vi "Subpanel PoC.vi"() -> ()   [LabVIEW 2021]
uses:
  <vilib>/Utility/LVLibp/NI_PackedLibraryUtility.lvlib
panel:
  in  "stop":bool
  out "qualified names":string[](array[string])
  out "error out":errorcluster
  in  "vi path":path=path "D:/dev/builds/TemplatePlugin/UI/CIF_Template_UI.lvlibp"
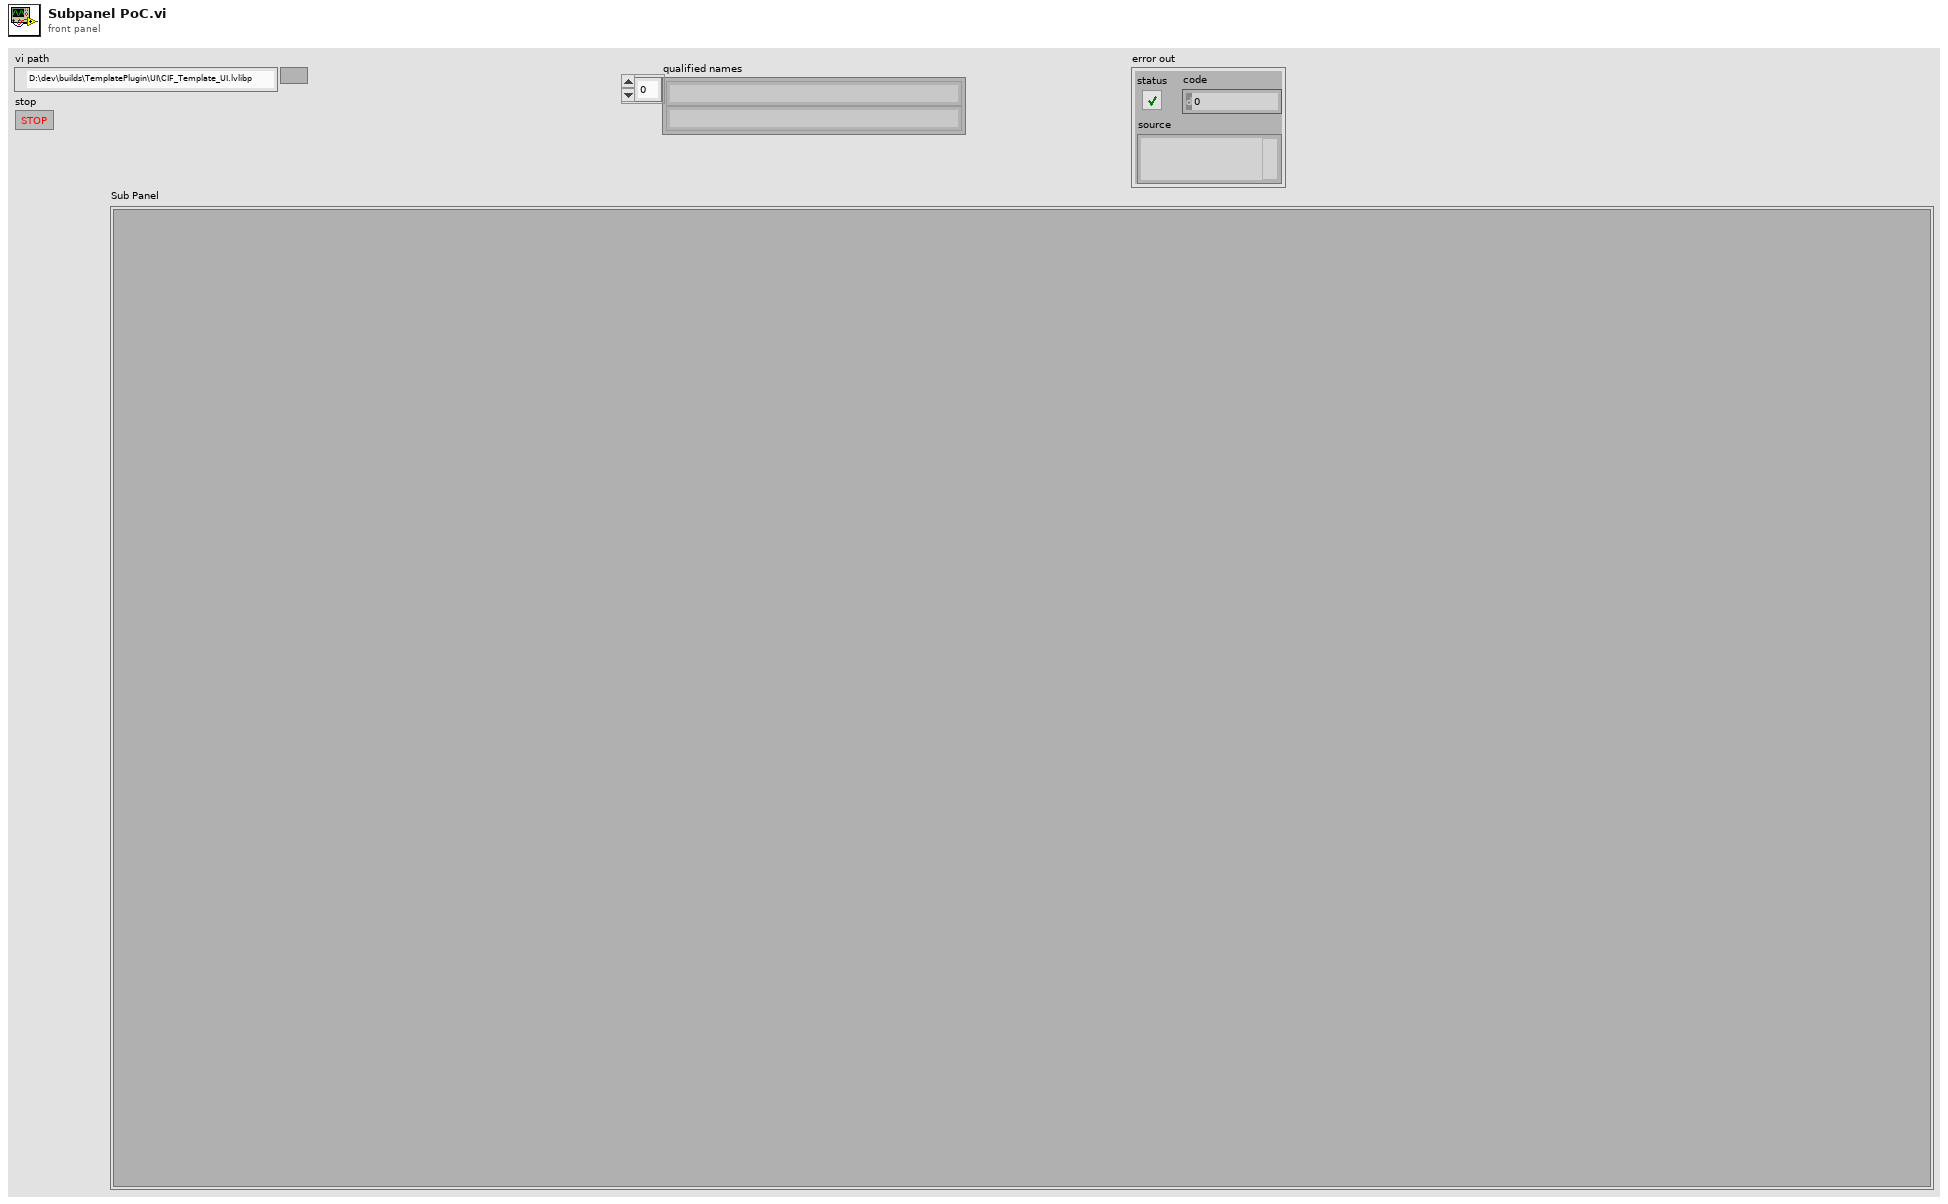
[diagram p1: front panel]
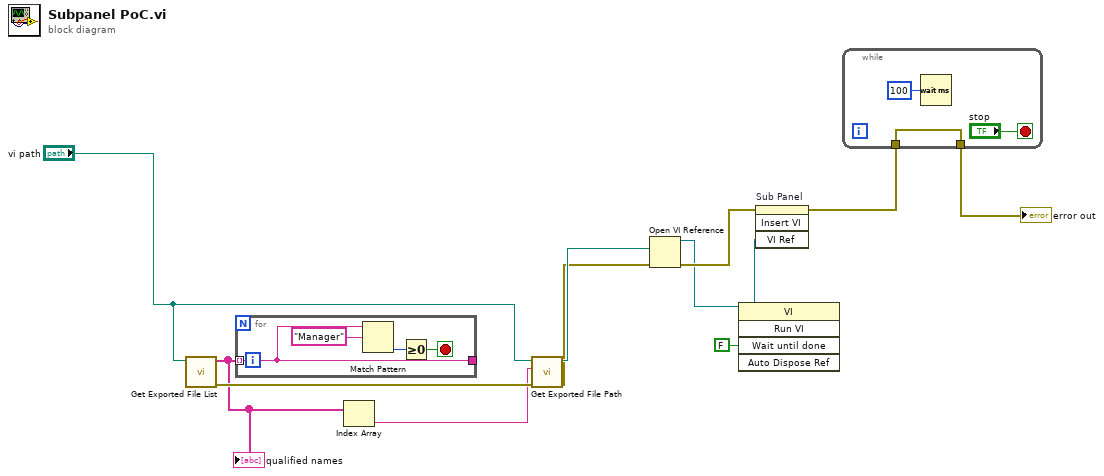
[diagram p0: block diagram]
diagram:
  n1 = call <vilib>:"Get Exported File List.vi"("packed library path"="vi path") -> ("error out"=w12:errorcluster, "qualified names"=w7:string[])  [unwired: 8 in, 1 out]
  "qualified names" <- w7
  n2 = for {
    tunnel: w7 -> [w13] mode=indexing
    tunnel: [w13] -> _
    stop <- w15 stop-if-true
    n3 = Match Pattern(string=w13, regular expression="Manager") -> (offset past match=w16:i32)  [unwired: 1 in, 3 out]
    n4 = Greater Or Equal To 0?(x=w16) -> (x >= 0?=w15:bool)
  }
  n5 = Index Array(array=w7) -> (element=w6:string)  [unwired: 1 in]
  n6 = call <vilib>:"Get Exported File Path.vi"("error in (no error)"=w12, "qualified name"=w6, "packed library path"="vi path") -> ("error out"=w9:errorcluster, "path"=w10:path)  [unwired: 7 in]
  n7 = Open VI Reference(vi path=w10, error in (no error)=w9) -> (vi reference=w5:refnum<vi>, error out=w8:errorcluster)  [unwired: 4 in]
  n8 = invoke class="VI" method="Run VI"(reference=w5, "Wait until done"=FALSE ("Wait Until Done")) -> (reference out=w4:refnum<vi>)  [unwired: 3 in, 4 out]
  n9 = invoke on="Sub Panel" class="SubPnl" method="Insert VI"(error in=w8, "VI Ref"=w4) -> (error out=w2:errorcluster)  [unwired: 2 in, 3 out]
  n10 = while {
    tunnel: [w19] -> w1
    tunnel: w2 -> [w19]
    stop <- "stop" stop-if-true
    n11 = Wait (ms)(milliseconds to wait=u32 100) -> ()  [unwired: 1 out]
  }
  "error out" <- w1
